vi "ESP_UDP_Rezero.vi"() -> ()   [LabVIEW 2021]
panel:
  in  "Re-zero":bool
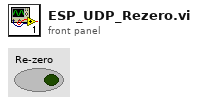
[diagram p1: front panel]
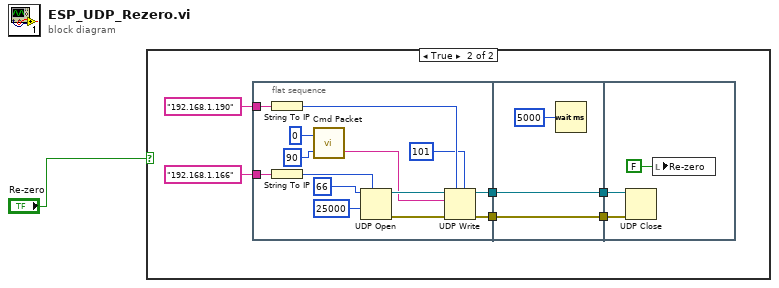
[diagram p0: block diagram]
diagram:
  n1 = case shown="True" "Re-zero" {
    frame False {
    }
    frame True {
      n2 = flat-sequence {
        tunnel: "192.168.1.166" ("Hardware Trigger") -> [w17]
        tunnel: "192.168.1.190" ("IP address") -> [w13]
        tunnel: [w9] -> w7
        tunnel: [w8] -> w6
        tunnel: [w23] -> w5
        tunnel: w7 -> [w23]
        tunnel: [w22] -> w4
        tunnel: w6 -> [w22]
        tunnel: w5 -> [w27]
        tunnel: w4 -> [w26]
        frame #0 {
          n3 = String To IP(1:w13) -> (0:w19:u32)
          n4 = String To IP(1:w17) -> (0:w16:u32)
          n5 = call "Cmd Packet.vi"("Command Byte"=90 ("data in"), "Parameter Byte"=0 ("data in")) -> ("Command Packet Byte String"=w10:string)  [unwired: 1 out]
          n6 = UDP Open(7:w16, 9:25000 ("timeout ms (60000)"), 11:u16 66 ("port")) -> (port=w20:refnum<k16>, 0:w21:errorcluster)  [unwired: 2 in, 1 out]
          n7 = UDP Write(address=w19, port or service name=u16 101 ("Port"), connection ID=w20, data in=w10, 8:w21) -> (error out=w9:errorcluster, 3:w8:refnum<k16>)  [unwired: 1 in]
        }
        frame #1 {
          n8 = Wait (ms)(milliseconds to wait=u32 5000) -> ()  [unwired: 1 out]
        }
        frame #2 {
          n9 = UDP Close(connection ID=w26, 8:w27) -> ()  [unwired: 2 out]
          n10 = local write "Re-zero"(FALSE) -> ()
        }
      }
    }
  }
